vi "Error Handler.vi"(7 "function":T1=enum."chown", 8 "error in (no error)":errorcluster, 11 "errno":i32) -> (0 "error out":errorcluster)   [LabVIEW 2013, in "Linux RT Utilities.lvlib"]
uses:
  Linux RT Utilities.lvlib
  Controls/Private/c functions.ctl
  <vilib>/NI/NI Linux RT Errno/Controls/Public/errno.ctl
  <vilib>/NI/NI Linux RT Errno/Linux Errno.lvlib
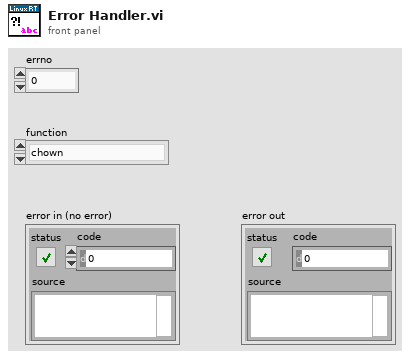
[diagram p1: front panel]
types:
  T1 = typedef "Linux RT Utilities.lvlib/c functions.ctl" = enum16{"unspecified", "chown", "fchown", "chmod", "fchmod"}
  T2 = typedef "Linux Errno.lvlib/errno.ctl" = enum16{"NONE", "EPERM", "ENOENT", "ESRCH", "EINTR", "EIO", "ENXIO", "E2BIG", "ENOEXEC", "EBADF", "ECHILD", "EAGAIN", "ENOMEM", "EACCES", "EFAULT", "ENOTBLK", "EBUSY", "EEXIST", "EXDEV", "ENODEV", "ENOTDIR", "EISDIR", "EINVAL", "ENFILE", "EMFILE", "ENOTTY", "ETXTBSY", "EFBIG", "ENOSPC", "ESPIPE", "EROFS", "EMLINK", "EPIPE", "EDOM", "ERANGE", "EDADLK", "ENAMETOOLONG", "ENOLCK", "ENOSYS", "ENOTEMPTY", "ELOOP", "EWOULDBLOCK", "ENOMSG", "EIDRM", "ECHRNG", "EL2NSYNC", "EL3HLT", "EL3RST", "ELNRNG", "EUNATCH", "ENOCSI", "EL2HLT", "EBADE", "EBADR", "EXFULL", "ENOANO", "EBADRQC", "EBADSLT", "EDEADLOCK", "EBFONT", "ENOSTR", "ENODATA", "ETIME", "ENOSR", "ENONET", "ENOPKG", "EREMOTE", "ENOLINK", "EADV", "ESRMNT", "ECOMM", "EPROTO", "EMULTIHOP", "EDOTDOT", "EBADMSG", "EOVERFLOW", "ENOTUNIQ", "EBADFD", "EREMCHG", "ELIBACC", "ELIBBAD", "ELIBSCN", "ELIBMAX", "ELIBEXEC", "ELISEQ", "ERESTART", "ESTRPIPE", "EUSERS", "ENOTSOCK", "EDESTADDRREQ", "EMSGSIZE", "EPROTOTYPE", "ENOPROTOOPT", "EPROTONOSUPPORT", "ESOCKTNOSUPPORT", "EOPNOTSUPP", "EPFNOSUPPORT", "EAFNOSUPPORT", "EADDRINUSE", "EADDRNOTAVAIL", "ENETDOWN", "ENETUNREACH", "ENETRESET", "ECONNABORTED", "ECONNRESET", "ENOBUFS", "EISCONN", "ENOTCONN", "ESHUTDOWN", "ETOOMANYREFS", "ETIMEDOUT", "ECONNREFUSED", "EHOSTDOWN", "EHOSTUNREACH", "EALREADY", "EINPROGRESS", "ESTALE", "EUCLEAN", "ENOTNAM", "ENAVAIL", "EISNAM", "EREMOTEIO", "EDQUOT", "ENOMEDIUM", "EMEDIUMTYPE", "ECANCELED", "ENOKEY", "EKEYEXPIRED", "EKEYREVOKED", "EKEYREJECTED", "EOWNERDEAD", "ENOTRECOVERABLE", "UNDEFINED"}
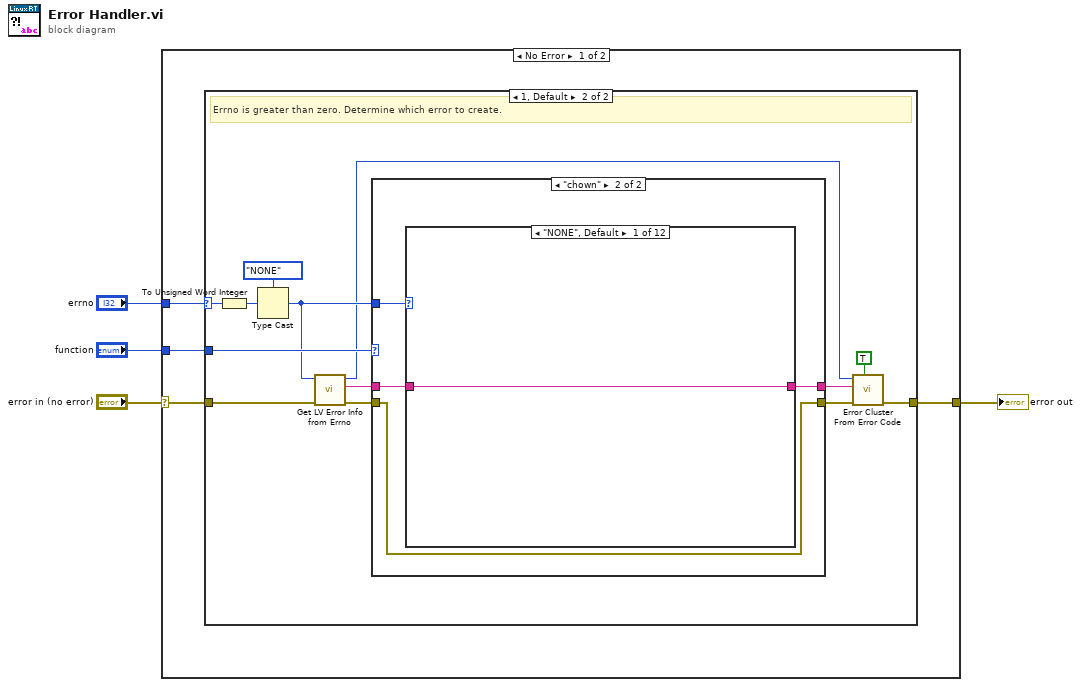
[diagram p0: block diagram]
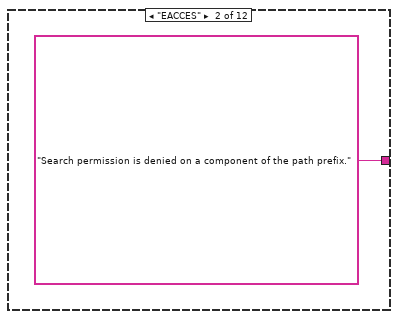
[diagram p4: hidden frame]
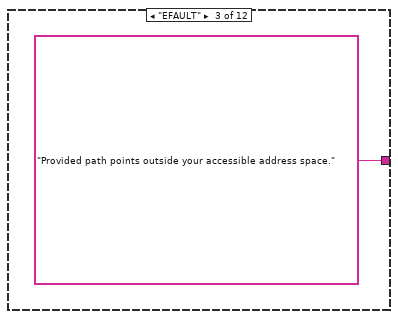
[diagram p5: hidden frame]
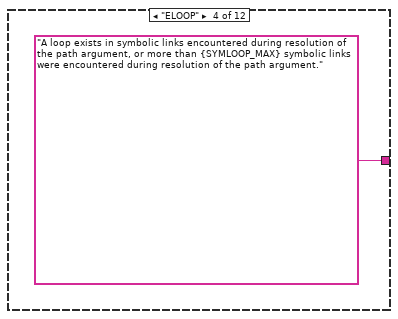
[diagram p6: hidden frame]
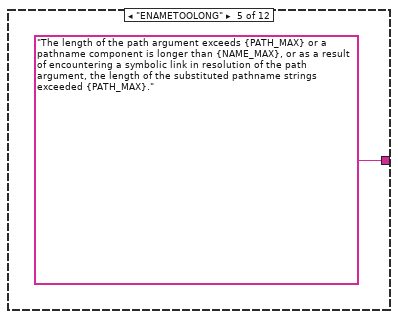
[diagram p7: hidden frame]
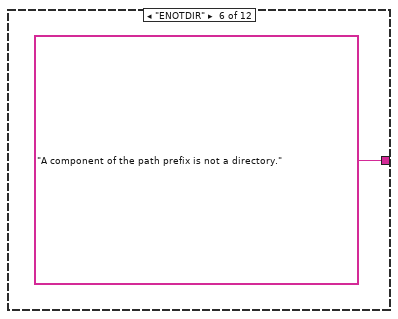
[diagram p8: hidden frame]
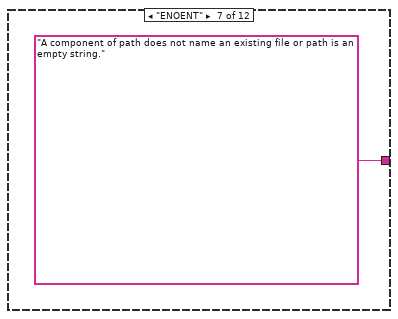
[diagram p9: hidden frame]
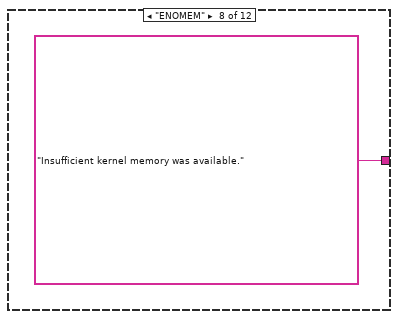
[diagram p10: hidden frame]
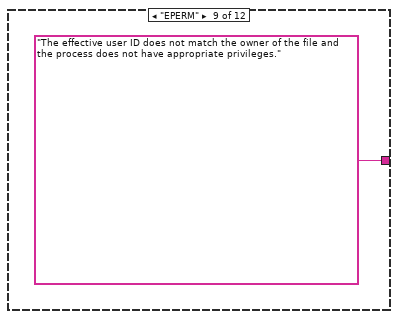
[diagram p11: hidden frame]
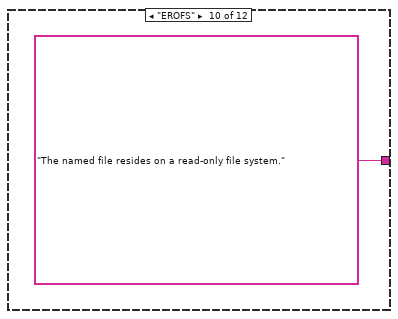
[diagram p12: hidden frame]
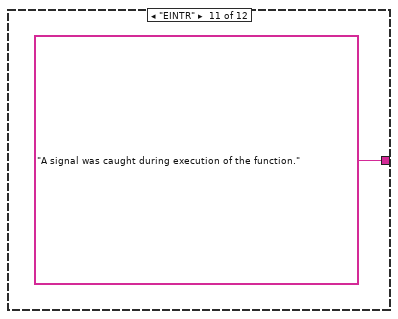
[diagram p13: hidden frame]
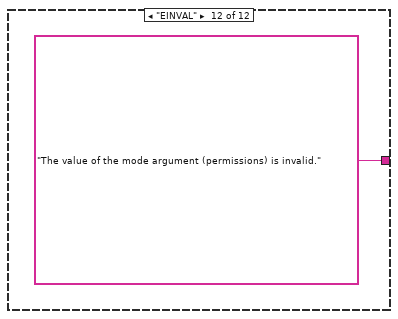
[diagram p14: hidden frame]
diagram:
  n1 = case shown="No Error" "error in (no error)" {
    selector: "error in (no error)" -> [w6 w41]
    tunnel: [w8 w41] -> w3
    tunnel: "errno" -> [w5 _]
    tunnel: "function" -> [w7 _]
    frame No Error {
      n2 = case shown="1, Default" w5 {
        selector: w5 -> [_ w15]
        tunnel: [w9 w22] -> w8
        tunnel: w7 -> [_ w20]
        tunnel: w6 -> [w9 w14]
        frame 0 {
          # "Errno is zero. No error occurred."
        }
        frame 1, Default {
          # "Errno is greater than zero. Determine which error to create."
          n3 = To Unsigned Word Integer(number=w15) -> (unsigned 16bit integer=w18:u16)
          n4 = Type Cast(type=errno."NONE" ("errno"), x=w18) -> (*(type *) &x=w12:T2)
          n5 = call <vilib>:"Get LV Error Info from Errno.vi"("error in (no error)"=w14, "errno"=w12) -> ("error out"=w13:errorcluster, "error description"=w10:string, "error code"=w11:i32)  [unwired: 7 in]
          n6 = case shown="\"chown\"" w20 {
            tunnel: w12 -> [_ w28]
            tunnel: [w23 w27] -> w19
            tunnel: w13 -> [w24 w26]
            tunnel: [w24 w26] -> w16
            tunnel: w10 -> [w23 w25]
            frame "unspecified", Default {
              # "No specific function was specified, so use generic error description."
            }
            frame "chown" {
              n7 = case shown="\"NONE\", Default" w28 {
                tunnel: [w29 "Search permission is denied on a component of the path prefix." "Provided path points outside your accessible address space." "A loop exists in symbolic links encountered during resolution of the path argument, or more than {SYMLOOP_MAX} symbolic links were encountered during resolution of the path argument." "The length of the path argument exceeds {PATH_MAX} or a pathname component is longer than {NAME_MAX}, or as a result of encountering a symbolic link in resolution of the path argument, the length of the substituted pathname strings exceeded {PATH_MAX}." "A component of the path prefix is not a directory." "A component of path does not name an existing file or path is an empty string." "Insufficient kernel memory was available." "The effective user ID does not match the owner of the file and the process does not have appropriate privileges." "The named file resides on a read-only file system." "A signal was caught during execution of the function." "The value of the mode argument (permissions) is invalid."] -> w27
                tunnel: w25 -> [w29 _ _ _ _ _ _ _ _ _ _ _]
                frame "NONE", Default {
                }
                frame "EACCES" {
                }
                frame "EFAULT" {
                }
                frame "ELOOP" {
                }
                frame "ENAMETOOLONG" {
                }
                frame "ENOTDIR" {
                }
                frame "ENOENT" {
                }
                frame "ENOMEM" {
                }
                frame "EPERM" {
                }
                frame "EROFS" {
                }
                frame "EINTR" {
                }
                frame "EINVAL" {
                }
              }
            }
          }
          n8 = call <vilib>:"Error Cluster From Error Code.vi"("show call chain? (False)"=TRUE, "error in (no error)"=w16, "error message (\"\")"=w19, "error code (0)"=w11) -> ("error out"=w22:errorcluster)  [unwired: 5 in]
        }
      }
    }
    frame Error {
      # "Error already exists. Pass through."
    }
  }
  "error out" <- w3
